vi "UpdateFFTgraphSequence.vi"() -> ()   [LabVIEW 2015]
panel:
  out "Intensity Graph":dbl[][](graph)
  out "NbX max":dbl
  out "NbZ max":dbl
  in  "disabled index (col)":i32
  out "subarray":dbl[](array[numeric])
  in  "logfile":string[][](array[string])
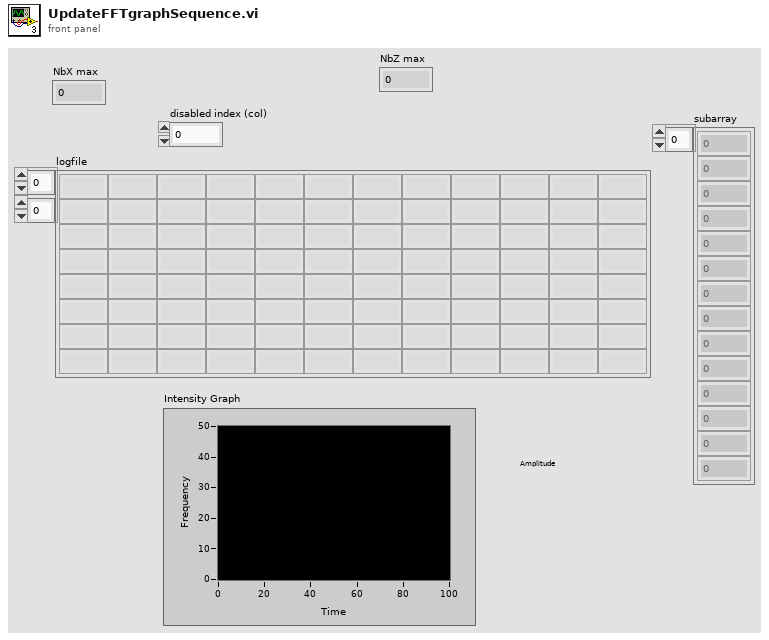
[diagram p1: front panel]
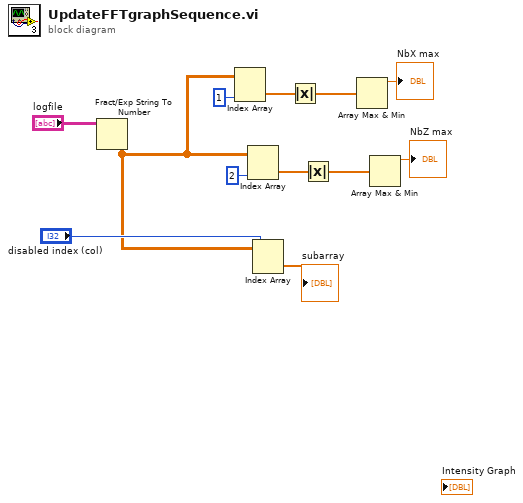
[diagram p0: block diagram]
diagram:
  n1 = Fract/Exp String To Number(string="logfile") -> (number=w1:dbl[][])  [unwired: 3 in, 1 out]
  n2 = Index Array(array=w1, index (col)=1 ("disabled index (col)")) -> (element=w4:dbl[])  [unwired: 1 in]
  n3 = Index Array(array=w1, index (col)=2 ("disabled index (col)")) -> (element=w8:dbl[])  [unwired: 1 in]
  n4 = Index Array(array=w1, index (col)="disabled index (col)") -> (element=→"subarray":dbl[])  [unwired: 1 in]
  n5 = Absolute Value(x=w4) -> (abs(x)=w3:dbl[])
  n6 = Absolute Value(x=w8) -> (abs(x)=w7:dbl[])
  n7 = Array Max & Min(array=w3) -> (max value=→"NbX max":dbl)  [unwired: 3 out]
  n8 = Array Max & Min(array=w7) -> (max value=→"NbZ max":dbl)  [unwired: 3 out]
